vi "PCA9525 - Read.vi"(0 "Handle In":u64, 5 "deviceAddress":u8, 7 "buffer":u8[](array[numeric])=[2, 0, 0], 11 "error in (no error)":errorcluster) -> (4 "handle":u64 format="%x", 6 "buffer out":u8[](array[numeric]), 8 "sizeTransferred":u32, 10 "pass?":bool, 15 "error out":errorcluster)   [LabVIEW 2024]
doc: "C command for reading the PCA9535 using I2C."
uses:
  I2C/libMPSSE-I2C.lvlib
  libmpsse.dll
panel:
  out "return type":u64
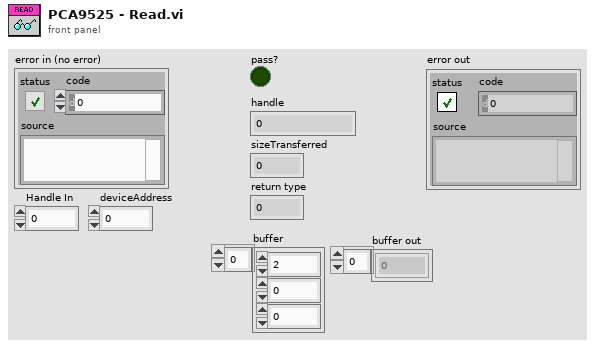
[diagram p1: front panel]
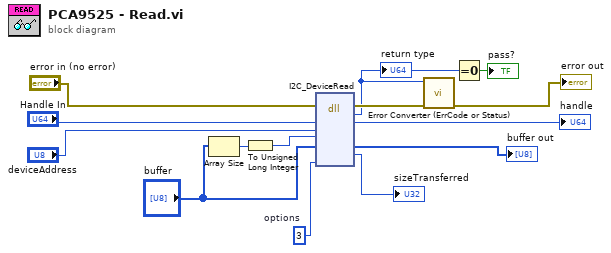
[diagram p0: block diagram]
diagram:
  w10 = u32 3  # options
  n1 = Array Size(array="buffer") -> (size(s)=w4:i32)
  n2 = To Unsigned Long Integer(number=w4) -> (unsigned 32bit integer=w2:u32)
  n3 = dll-call lib="libmpsse.dll" fn="I2C_DeviceRead"(error in="error in (no error)", "handle"="Handle In", "deviceAddress"="deviceAddress", "sizeToTransfer"=w2, "buffer"="buffer", "options"=w10) -> (error out=w9:errorcluster, "return type"=w8:u64, "handle"=→"handle":u64, "buffer"=→"buffer out":u8[], "sizeTransferred"=→"sizeTransferred":u32)  [unwired: 6 in, 1 out]
  "return type" <- w8
  n4 = call "Error Converter (ErrCode or Status).vi"("error in (no error)"=w9, "error code"=w8) -> ("error out"=→"error out":errorcluster)  [unwired: 9 in]
  n5 = Equal To 0?(x=w8) -> (x = 0?=→"pass?":bool)
